vi "Modified Bessel Function Kn.vi"(2 "n":i32, 3 "x":dbl format="%.2f") -> (1 "Kn(x)":dbl format="%.2f")   [LabVIEW 2020, in "NI_Gmath.lvlib"]
doc: "Computes the modified Bessel function of the second kind."
uses:
  NI_Gmath.lvlib
  <resource>/lvanlys.dll
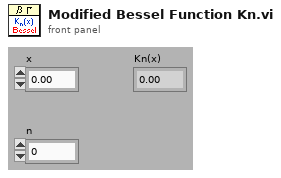
[diagram p1: front panel]
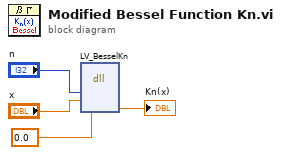
[diagram p0: block diagram]
diagram:
  n1 = dll-call lib="C:/Program Files (x86)/National Instruments/LabVIEW 2020/resource/lvanlys.*" fn="LV_BesselKn"("n"="n", "x"="x", "Kn(x)"=0.0 ("Jr")) -> ("Kn(x)"=→"Kn(x)":dbl)  [unwired: 6 in, 2 out]
